vi "PressureSensor.vi"(7 "Action":T4, 8 "error in (no error)":errorcluster, 10 "PressureScaler":dbl=1.0, 11 "AIDeviceRef":T1={"DevStatus"={"status"=FALSE, "code"=0, "source"=""}, "Analog Module"=enum."Analog Module 1", "Analog Channel"=enum."Invalid"}) -> (0 "error out":errorcluster, 3 "Pressure":dbl)   [LabVIEW 2013]
uses:
  PressureSensorAction.ctl
  <vilib>/Rock Robotics/WPI/AnalogChannel/WPI_AnalogChannelDevRef.ctl
  <vilib>/Rock Robotics/SystemInterfaces/Typedef/FPGA_TypedefAnalogModule.ctl
  <vilib>/Rock Robotics/SystemInterfaces/AI/FPGA_AIChannel.ctl
panel:
  in  "Samples Per Second":dbl=1000.0
  in  "AverageBits":u8=3
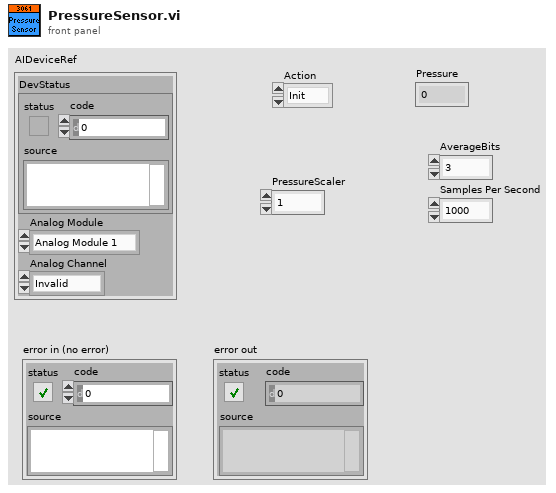
[diagram p1: front panel]
types:
  T1 = typedef "WPI_AnalogChannelDevRef.ctl" = cluster{"DevStatus":errorcluster, "Analog Module":T2, "Analog Channel":T3}
  T2 = typedef "FPGA_TypedefAnalogModule.ctl" = enum16{"Analog Module 1", "Analog Module 2"}
  T3 = typedef "FPGA_AIChannel.ctl" = enum8{"AI 1", "AI 2", "AI 3", "AI 4", "AI 5", "AI 6", "AI 7", "AI 8", "Invalid"}
  T4 = typedef "PressureSensorAction.ctl" = enum16{"Init", "ReadValue", "Disable"}
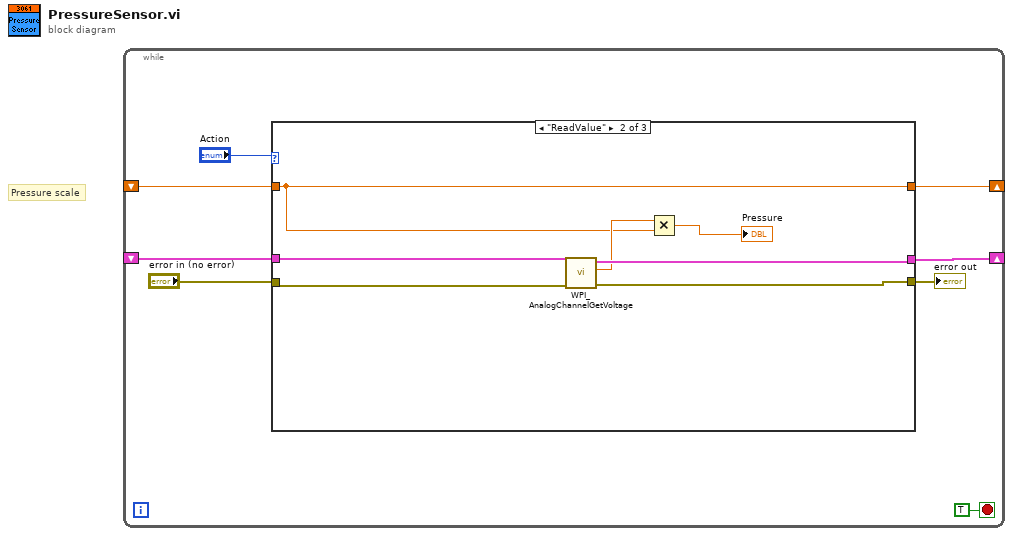
[diagram p0: block diagram]
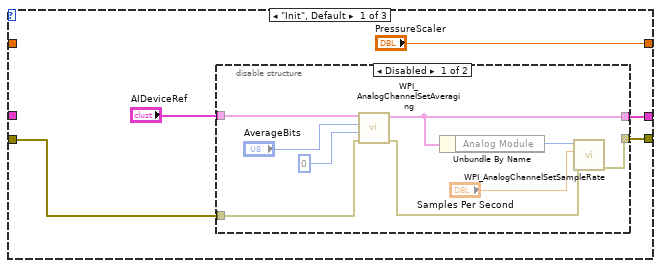
[diagram p2: hidden frame]
diagram:
  # "Pressure scale"
  n1 = while {
    shift-right: [w7] -> _
    shift-left: _ -> [w6]
    shift-right: [w2] -> _
    shift-left: _ -> [w1]
    stop <- TRUE stop-if-true
    n2 = case shown="\"ReadValue\"" "Action" {
      tunnel: [w12 w28 w32] -> w7
      tunnel: w6 -> [_ w29 w32]
      tunnel: "error in (no error)" -> [w11 w25 w31]
      tunnel: [w10 w24 w31] -> w4
      tunnel: ["PressureScaler" w23 w30] -> w2
      tunnel: w1 -> [_ w23 w30]
      frame "Init", Default {
        n3 = disable-structure shown="Disabled" {
          disable-tunnel: "AIDeviceRef" -> [w22 _]
          disable-tunnel: [w21 _] -> w12
          disable-tunnel: w11 -> [w16 _]
          disable-tunnel: [w14 _] -> w10
          frame Disabled {
            n4 = call <vilib>:"WPI_AnalogChannelSetAveraging.vi"("error in (no error)"=w16, "OversampleBits"=u8 0, "AverageBits"="AverageBits", "AIDeviceRef"=w22) -> ("error out"=w15:errorcluster, "AIDeviceRef"=w21:T1)  [unwired: 6 out]
            n5 = Unbundle By Name(w21) -> ("Analog Module"=w20:T2)
            n6 = call <vilib>:"WPI_AnalogChannelSetSampleRate.vi"("error in (no error)"=w15, "Samples Per Second"="Samples Per Second", "Analog Module (Module 1)"=w20) -> ("error out"=w14:errorcluster)  [unwired: 1 in, 7 out]
          }
          frame Enabled {
          }
        }
      }
      frame "ReadValue" {
        n7 = call <vilib>:"WPI_AnalogChannelGetVoltage.vi"("error in (no error)"=w25, "AIDeviceRef"=w29) -> ("error out"=w24:errorcluster, "Voltage"=w27:dbl, "AIDeviceRef"=w28:T1)  [unwired: 7 in]
        n8 = Multiply(x=w27, y=w23) -> (x*y=→"Pressure":dbl)
      }
      frame "Disable" {
      }
    }
    "error out" <- w4
  }
